vi "RSZVB Configure Trigger Free Run.vi"(8 "error in (no error)":errorcluster {"code" format="%.0x"}, 10 "Channel (1)":i32=1, 11 "VISA session":refnum<visa-resource-name>) -> (0 "error out":errorcluster {"code" format="%.0x"}, 3 "dup VISA session":refnum<visa-resource-name>)   [LabVIEW 2011]
doc: "This VI configures free run measurement without waiting for trigger events.\n\nRemote-control command(s):\nTRIGger<Ch>[:SEQuence]:SOURce IMMediate"
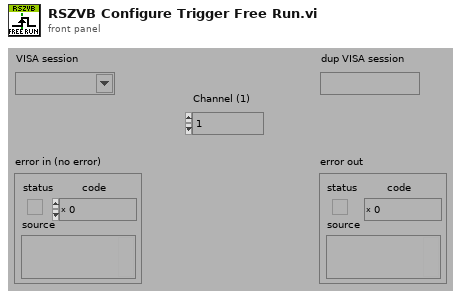
[diagram p1: front panel]
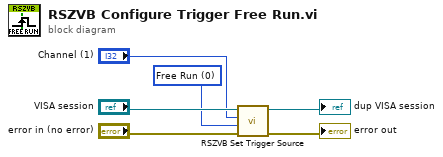
[diagram p0: block diagram]
diagram:
  w1 = 0 items=["Free Run", "External", "Periodic", "Manual", "RF Power"] ("Trigger Source (0: Free Run)")
  n1 = call "RSZVB Set Trigger Source.vi"("error in (no error)"="error in (no error)", "Trigger Source (0: Free Run)"=w1, "Channel (1)"="Channel (1)", "VISA session"="VISA session") -> ("error out"=→"error out":errorcluster, "dup VISA session"=→"dup VISA session":refnum<visa-resource-name>)  [unwired: 6 in]
